vi "New.vi"(10 "note refnum":refnum<vi>, 11 "title refnum":refnum<vi>) -> ()   [LabVIEW 2020]
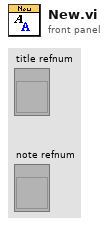
[diagram p1: front panel]
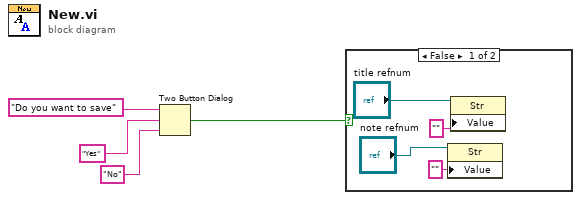
[diagram p0: block diagram]
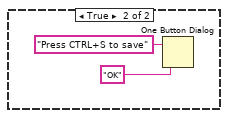
[diagram p2: hidden frame]
diagram:
  n1 = Two Button Dialog(message="Do you want to save", 1:"No" ("F button name (\"Cancel\")"), 2:"Yes" ("T button name (\"OK\")")) -> (T button?=w4:bool)
  n2 = case shown="False" w4 {
    frame False {
      n3 = property class="Str"(reference="note refnum", "Value"="") -> ()  [unwired: 1 in, 2 out]
      n4 = property class="Str"(reference="title refnum", "Value"="") -> ()  [unwired: 1 in, 2 out]
    }
    frame True {
      n5 = One Button Dialog(message="Press CTRL+S to save", button name ("OK")="OK") -> ()  [unwired: 1 out]
    }
  }
